vi "main.vi"() -> ()   [LabVIEW 2020]
uses:
  defTypeConfigs/mainConfigs.ctl
  defTypeConfigs/spectroConfig.ctl
  defTypeConfigs/tempConfig.ctl
  defTypeConfigs/expConfig.ctl
panel:
  out "mainConfigs":T1={"spectroConfig"={"Grating"=0, "waveLength"=0, "sampleTime"=0.0, "nbStrip"=0, "gap"=0, "Background path"=path "", "temperature"=0.0, "binning"=0, "Camera handle"=0, "Spectro handle"=0, "Xdim"=0, "Ydim"=0}, "tempConfig"={"ComPort"="COM4", "SensorNumber"=1.0, "PID"={"P"=0.0, "I"=0.0, "D"=0.0}}, "expConfig"={"colorParameters"={"giver"="", "acceptor"=[]}, "recordDataInTDMS?"=TRUE, "PID_mode"=enum."rampe"}}
  in  "Experience parameters":bool caption="Check experience parameters"
  out "Background out path":path
  out "TDMS file out path":path
  in  "PathsConfig setup":bool caption="Application paths"
  in  "Read acquisition":bool
  out "message":string
  out "configsIsOKCluster":T5
  out "Error OUT":errorcluster caption="constante d'erreur"
  in  "Error IN":errorcluster caption="constante d'erreur"
  in  "Kill app":bool
  in  "TempConfig setup":bool caption="Temp config is OK"
  in  "SpectroConfig setup":bool caption="Check spectro config"
  in  "Start Acquisition":bool
  # "RADIO PROJECT\nAPPLICATION"
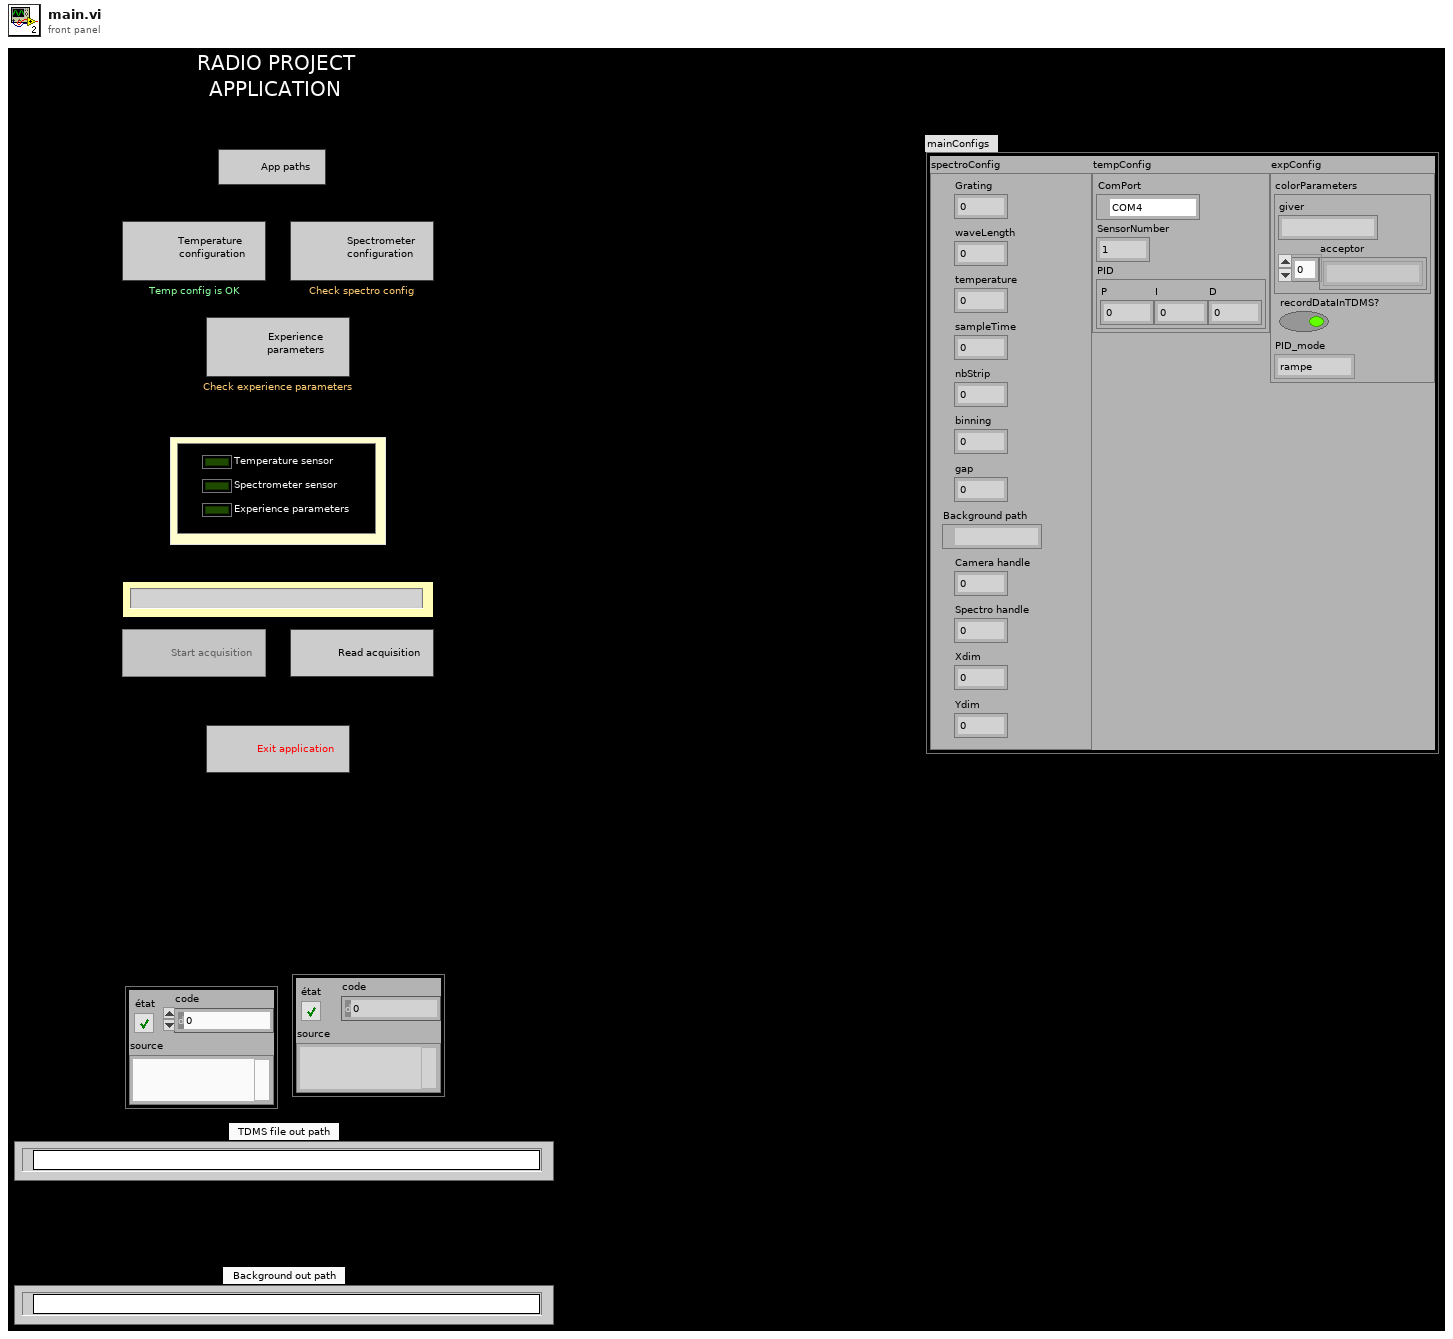
[diagram p1: front panel]
types:
  T1 = typedef "mainConfigs.ctl" = cluster{"spectroConfig":T2, "tempConfig":T3, "expConfig":T4}
  T2 = typedef "spectroConfig.ctl" = cluster{"Grating":i32, "waveLength":i32, "sampleTime":dbl, "nbStrip":i32, "gap":i32, "Background path":path, "temperature":dbl, "binning":i32, "Camera handle":i32, "Spectro handle":i32, "Xdim":i32, "Ydim":i32}
  T3 = typedef "tempConfig.ctl" = cluster{"ComPort":refnum<visa-resource-name>, "SensorNumber":dbl, "PID":cluster{"P":dbl, "I":dbl, "D":dbl}}
  T4 = typedef "expConfig.ctl" = cluster{"colorParameters":cluster{"giver":string, "acceptor":string[]}, "recordDataInTDMS?":bool, "PID_mode":enum16{"rampe", "triangle", "sinus", "carré", "continu"}}
  T5 = cluster{"Temperature sensor":bool, "Spectrometer sensor":bool, "Experience parameters":bool}
  T6 = cluster{"spectroConfigOk?":bool, "tempConfigOk?":bool, "tempConfigOk? 2":bool}
  T7 = enum8{"Enabled", "Disabled", "Disabled and Grayed Out"}
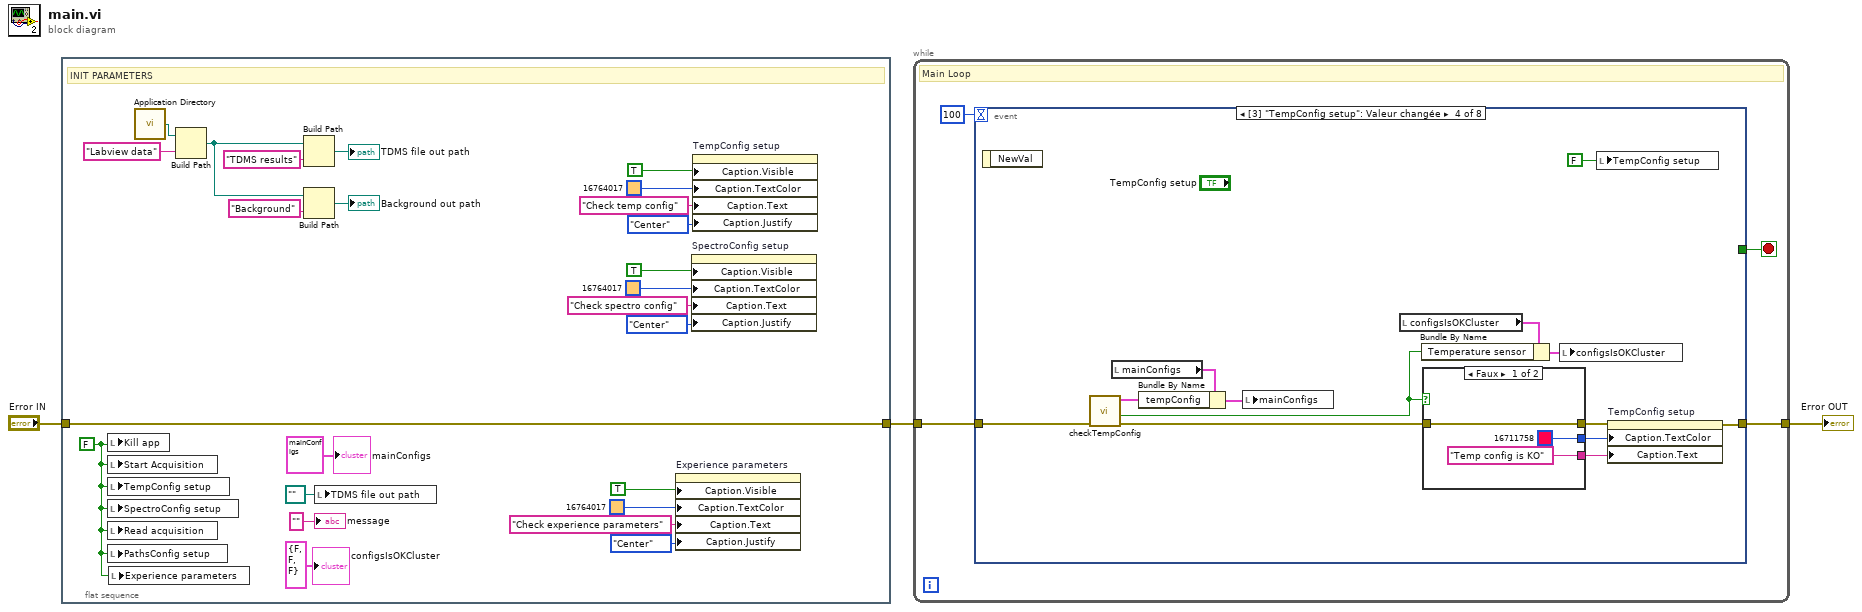
[diagram p0: block diagram]
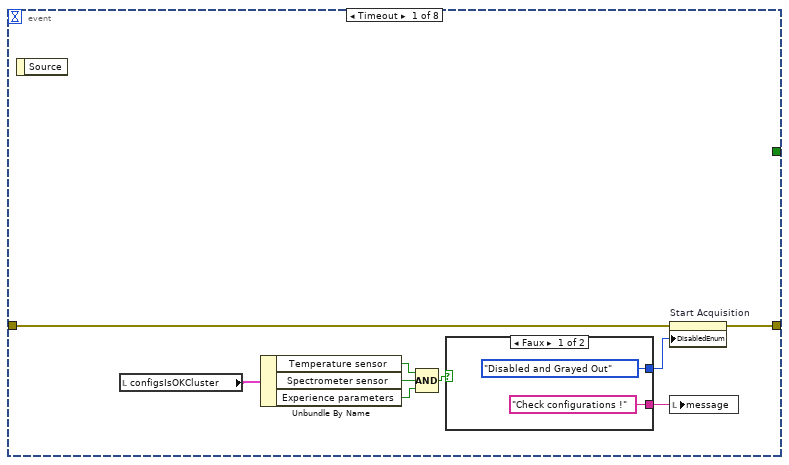
[diagram p2: hidden frame]
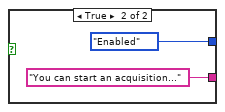
[diagram p3: hidden frame]
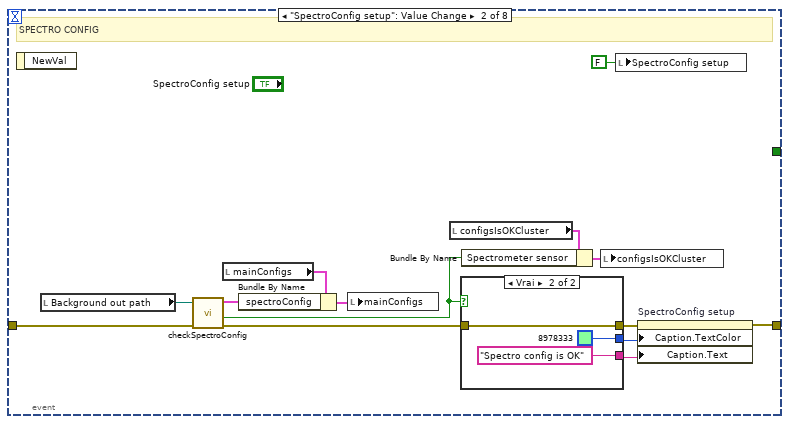
[diagram p4: hidden frame]
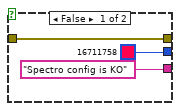
[diagram p5: hidden frame]
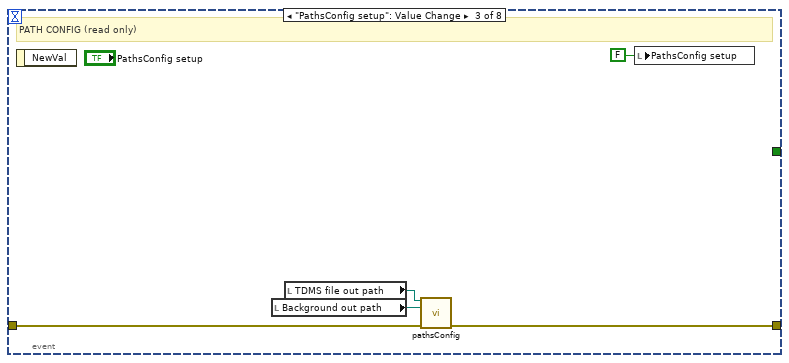
[diagram p6: hidden frame]
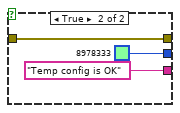
[diagram p7: hidden frame]
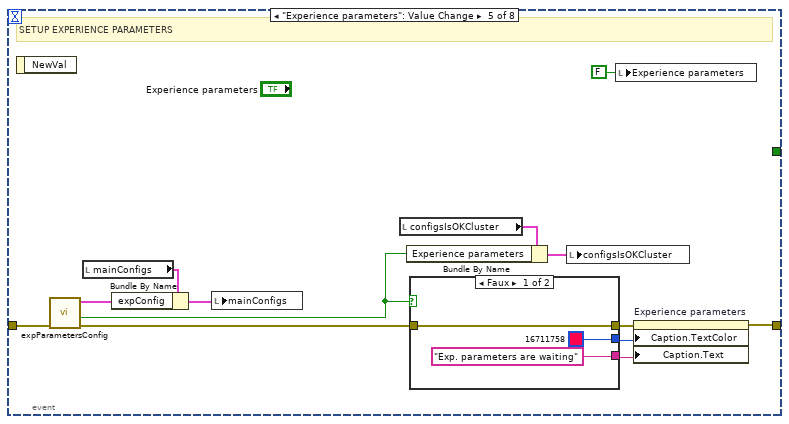
[diagram p8: hidden frame]
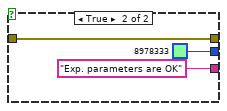
[diagram p9: hidden frame]
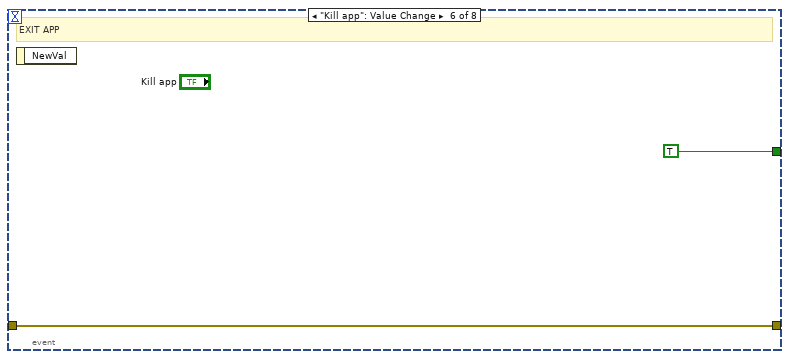
[diagram p10: hidden frame]
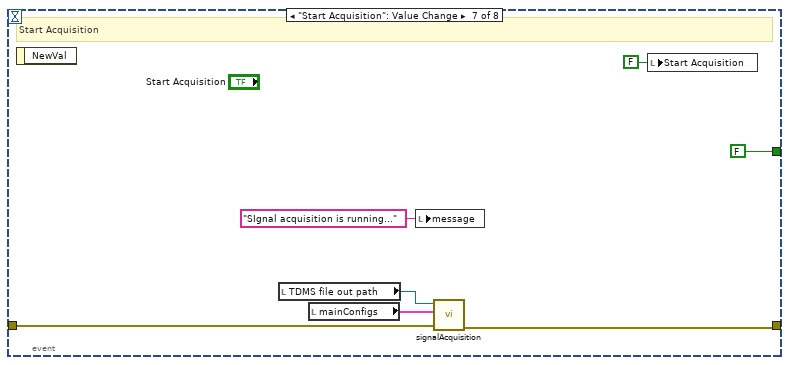
[diagram p11: hidden frame]
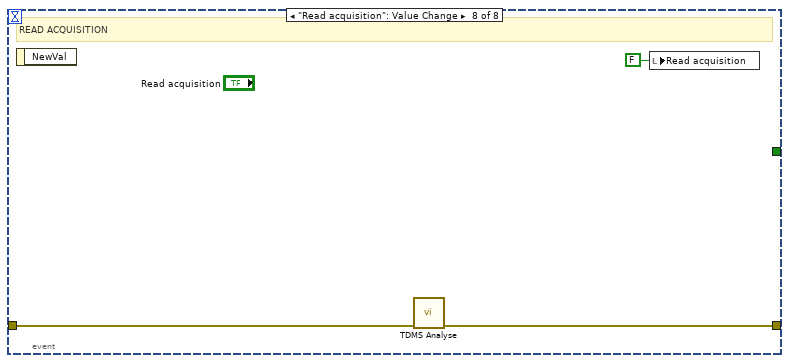
[diagram p12: hidden frame]
diagram:
  n1 = flat-sequence {
    tunnel: "Error IN" -> [w23]
    tunnel: [w23] -> w1
    frame #0 {
      w21 = FALSE ("Start Acquisition")
      # "INIT PARAMETERS"
      n2 = local write "Kill app"(w21) -> ()
      n3 = local write "Start Acquisition"(w21) -> ()
      n4 = local write "TempConfig setup"(w21) -> ()
      n5 = local write "SpectroConfig setup"(w21) -> ()
      n6 = local write "Read acquisition"(w21) -> ()
      n7 = local write "PathsConfig setup"(w21) -> ()
      n8 = local write "Experience parameters"(w21) -> ()
      n9 = call <vilib>:"Application Directory.vi"() -> ("Application Directory"=w26:path)
      n10 = Build Path(base path=w26, name or relative path="Labview data" ("nom ou chemin relatif")) -> (appended path=w4:path)
      n11 = Build Path(base path=w4, name or relative path="TDMS results" ("nom ou chemin relatif")) -> (appended path=→"TDMS file out path":path)
      n12 = Build Path(base path=w4, name or relative path="Background" ("nom ou chemin relatif")) -> (appended path=→"Background out path":path)
      n13 = local write "TDMS file out path"(path "" ("TDMS file out path")) -> ()
      n14 = property on="Experience parameters" class="Bool (strict)"("Caption.Visible"=TRUE ("Sous-titre.Visible"), "Caption.TextColor"=u32 16764017 ("Sous-titre.Couleurs du texte:Couleur du texte"), "Caption.Text"="Check experience parameters" ("Sous-titre.Texte"), "Caption.Justify"=enum16{"Left", "Center", "Right"}."Center" ("Sous-titre.Justification")) -> ()  [unwired: 2 in, 2 out]
      n15 = property on="SpectroConfig setup" class="Bool (strict)"("Caption.Visible"=TRUE ("Sous-titre.Visible"), "Caption.TextColor"=u32 16764017 ("Sous-titre.Couleurs du texte:Couleur du texte"), "Caption.Text"="Check spectro config" ("Sous-titre.Texte"), "Caption.Justify"=enum16{"Left", "Center", "Right"}."Center" ("Sous-titre.Justification")) -> ()  [unwired: 2 in, 2 out]
      n16 = property on="TempConfig setup" class="Bool (strict)"("Caption.Visible"=TRUE ("Sous-titre.Visible"), "Caption.TextColor"=u32 16764017 ("Sous-titre.Couleurs du texte:Couleur du texte"), "Caption.Text"="Check temp config" ("Sous-titre.Texte"), "Caption.Justify"=enum16{"Left", "Center", "Right"}."Center" ("Sous-titre.Justification")) -> ()  [unwired: 2 in, 2 out]
      "configsIsOKCluster" <- T6 {"spectroConfigOk?"=FALSE, "tempConfigOk?"=FALSE, "tempConfigOk? 2"=FALSE} ("configsIsOKCluster")
      "message" <- "" ("message")
      "mainConfigs" <- T1 {"spectroConfig"={"Grating"=0, "waveLength"=0, "sampleTime"=0.0, "nbStrip"=0, "gap"=0, "Background path"=path "", "temperature"=0.0, "binning"=0, "Camera handle"=0, "Spectro handle"=0, "Xdim"=0, "Ydim"=0}, "tempConfig"={"ComPort"="COM4", "SensorNumber"=1.0, "PID"={"P"=0.0, "I"=0.0, "D"=0.0}}, "expConfig"={"colorParameters"={"giver"="", "acceptor"=[]}, "recordDataInTDMS?"=TRUE, "PID_mode"=enum."rampe"}} ("mainConfigs")
    }
  }
  n17 = while {
    tunnel: w1 -> [w31]
    tunnel: [w30] -> w3
    stop <- w29 stop-if-true
    # "Main Loop"
    n18 = event shown="[3] \"TempConfig setup\": Valeur changée" {
      selector: _ -> [_ _ _ _ _ _ _ _]
      dyn-events: _ -> [_ _ _ _ _ _ _ _]
      timeout: 100 -> [_ _ _ _ _ _ _ _]
      tunnel: w31 -> [w40 w59 w69 w82 w101 w110 w114 w118]
      tunnel: [w39 w52 w68 w77 w93 w110 w113 w119] -> w30
      tunnel: [_ _ _ _ _ TRUE FALSE _] -> w29
      event Timeout {
        n19 = event-data() -> ()  [unwired: 1 in, 1 out]
        n20 = local read "configsIsOKCluster"() -> (w38:T5)
        n21 = Unbundle By Name(w38) -> ("Temperature sensor"=w37:bool, "Spectrometer sensor"=w36:bool, "Experience parameters"=w33:bool)
        n22 = Compound Arithmetic op=AND ("Opérateur arithmétique")(w37, w36, w33) -> (w35:bool)
        n23 = case shown="Faux" w35 {
          tunnel: [T7."Disabled and Grayed Out" ("Désactivé") T7."Enabled" ("Désactivé")] -> w41
          tunnel: ["Check configurations !" ("message") "You can start an acquisition..." ("message")] -> w34
          frame False {
          }
          frame True {
          }
        }
        n24 = property on="Start Acquisition" class="Bool (strict)"(error in=w40, "DisabledEnum"=w41) -> (error out=w39:errorcluster)  [unwired: 1 in, 1 out]
        n25 = local write "message"(w34) -> ()
      }
      event "SpectroConfig setup": Value Change {
        # "SPECTRO CONFIG"
        n26 = event-data() -> ()  [unwired: 1 in, 1 out]
        n27 = local read "Background out path"() -> (w46:path)
        n28 = call "checkSpectroConfig.vi"("Error IN"=w59, "Background folder path"=w46) -> ("Error OUT"=w57:errorcluster, "spectroConfigIsOk?"=w50:bool, "spectroConfig"=w48:T2)  [unwired: 7 in]
        n29 = local read "mainConfigs"() -> (w47:T1)
        n30 = Bundle By Name(cluster=w47, "spectroConfig"=w48) -> (w49:T1)
        n31 = local write "mainConfigs"(w49) -> ()
        n32 = local read "configsIsOKCluster"() -> (w55:T5)
        n33 = case shown="Vrai" w50 {
          tunnel: [w62 w63] -> w51
          tunnel: w57 -> [w62 w63]
          tunnel: [u32 16711758 ("Sous-titre.Couleurs du texte:Couleur du texte") u32 8978333 ("Sous-titre.Couleurs du texte:Couleur du texte")] -> w54
          tunnel: ["Spectro config is KO" ("Sous-titre.Texte") "Spectro config is OK" ("Sous-titre.Texte")] -> w53
          frame False {
          }
          frame True {
          }
        }
        n34 = Bundle By Name(cluster=w55, "Spectrometer sensor"=w50) -> (w56:T5)
        n35 = local write "configsIsOKCluster"(w56) -> ()
        n36 = local write "SpectroConfig setup"(FALSE ("SpectroConfig setup")) -> ()
        n37 = property on="SpectroConfig setup" class="Bool (strict)"(error in=w51, "Caption.TextColor"=w54, "Caption.Text"=w53) -> (error out=w52:errorcluster)  [unwired: 1 in, 1 out]
      }
      event "PathsConfig setup": Value Change {
        # "PATH CONFIG (read only)"
        n38 = event-data() -> ()  [unwired: 1 in, 1 out]
        n39 = local read "Background out path"() -> (w66:path)
        n40 = local read "TDMS file out path"() -> (w67:path)
        n41 = call "pathsConfig.vi"("TDMS file out path IN"=w67, "Background out path IN"=w66, "Error IN"=w69) -> ("Error OUT"=w68:errorcluster)  [unwired: 12 in]
        n42 = local write "PathsConfig setup"(FALSE ("PathsConfig setup")) -> ()
      }
      event "TempConfig setup": Value Change {
        n43 = event-data() -> ()  [unwired: 1 in, 1 out]
        n44 = call "checkTempConfig.vi"("ERROR IN"=w82) -> ("ERROR OUT"=w80:errorcluster, "tempConfigIsOk?"=w75:bool, "tempConfig"=w73:T3)  [unwired: 8 in]
        n45 = local read "mainConfigs"() -> (w72:T1)
        n46 = Bundle By Name(cluster=w72, "tempConfig"=w73) -> (w74:T1)
        n47 = local write "mainConfigs"(w74) -> ()
        n48 = local read "configsIsOKCluster"() -> (w71:T5)
        n49 = Bundle By Name(cluster=w71, "Temperature sensor"=w75) -> (w83:T5)
        n50 = case shown="Faux" w75 {
          tunnel: w80 -> [w86 w87]
          tunnel: [w86 w87] -> w76
          tunnel: [u32 16711758 ("Sous-titre.Couleurs du texte:Couleur du texte") u32 8978333 ("Sous-titre.Couleurs du texte:Couleur du texte")] -> w79
          tunnel: ["Temp config is KO" ("Sous-titre.Texte") "Temp config is OK" ("Sous-titre.Texte")] -> w78
          frame False {
          }
          frame True {
          }
        }
        n51 = local write "configsIsOKCluster"(w83) -> ()
        n52 = local write "TempConfig setup"(FALSE ("SpectroConfig setup")) -> ()
        n53 = property on="TempConfig setup" class="Bool (strict)"(error in=w76, "Caption.TextColor"=w79, "Caption.Text"=w78) -> (error out=w77:errorcluster)  [unwired: 1 in, 1 out]
      }
      event "Experience parameters": Value Change {
        # "SETUP EXPERIENCE PARAMETERS"
        n54 = event-data() -> ()  [unwired: 1 in, 1 out]
        n55 = call "expParametersConfig.vi"("Error IN"=w101) -> ("Error OUT"=w96:errorcluster, "expParamsIsOK"=w94:bool, "expConfig"=w91:T4)  [unwired: 8 in]
        n56 = local read "mainConfigs"() -> (w90:T1)
        n57 = Bundle By Name(cluster=w90, "expConfig"=w91) -> (w92:T1)
        n58 = local write "mainConfigs"(w92) -> ()
        n59 = local read "configsIsOKCluster"() -> (w99:T5)
        n60 = Bundle By Name(cluster=w99, "Experience parameters"=w94) -> (w100:T5)
        n61 = case shown="Faux" w94 {
          tunnel: [u32 16711758 ("Sous-titre.Couleurs du texte:Couleur du texte") u32 8978333 ("Sous-titre.Couleurs du texte:Couleur du texte")] -> w98
          tunnel: ["Exp. parameters are waiting" ("Sous-titre.Texte") "Exp. parameters are OK" ("Sous-titre.Texte")] -> w97
          tunnel: w96 -> [w103 w106]
          tunnel: [w103 w106] -> w95
          frame False {
          }
          frame True {
          }
        }
        n62 = local write "configsIsOKCluster"(w100) -> ()
        n63 = local write "Experience parameters"(FALSE ("Experience parameters")) -> ()
        n64 = property on="Experience parameters" class="Bool (strict)"(error in=w95, "Caption.TextColor"=w98, "Caption.Text"=w97) -> (error out=w93:errorcluster)  [unwired: 1 in, 1 out]
      }
      event "Kill app": Value Change {
        # "EXIT APP"
        n65 = event-data() -> ()  [unwired: 1 in, 1 out]
      }
      event "Start Acquisition": Value Change {
        # "Start Acquisition"
        n66 = event-data() -> ()  [unwired: 1 in, 1 out]
        n67 = local read "TDMS file out path"() -> (w112:path)
        n68 = local read "mainConfigs"() -> (w111:T1)
        n69 = local write "message"("SIgnal acquisition is running..." ("message")) -> ()
        n70 = call "signalAcquisition.vi"("Error IN"=w114, "mainConfigs"=w111, "Répertoire de sortie du fichier TDMS"=w112) -> ("Error OUT"=w113:errorcluster)  [unwired: 6 in, 2 out]
        n71 = local write "Start Acquisition"(FALSE ("Start Acquisition")) -> ()
      }
      event "Read acquisition": Value Change {
        # "READ ACQUISITION"
        n72 = event-data() -> ()  [unwired: 1 in, 1 out]
        n73 = call "TDMS Analyse.vi"("Error IN"=w118) -> ("Error OUT"=w119:errorcluster)  [unwired: 10 in]
        n74 = local write "Read acquisition"(FALSE ("Read acquisition")) -> ()
      }
    }
  }
  "Error OUT" <- w3
